vi "create event queue.vi"(8 "error in":errorcluster, 10 "size":i32, 11 "module in":refnum<class "TBM module execution interface.lvclass">) -> (0 "error out":errorcluster, 3 "module out":refnum<class "TBM module execution interface.lvclass">)   [LabVIEW 2013, in "TBM module execution interface.lvclass"]
uses:
  TBM module execution interface.lvclass
  TBM module execution interface.lvclass/TBM module execution interface.ctl
  <vilib>/NI/Tag Bus/events/data bus events.lvlib
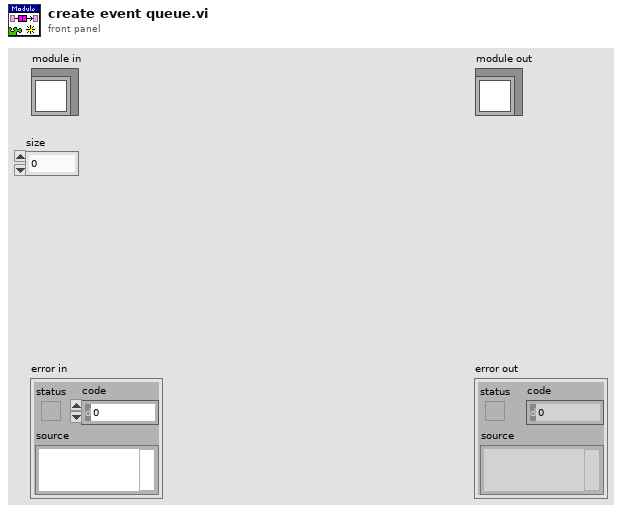
[diagram p1: front panel]
types:
  T1 = typedef "data bus events.lvlib/event queue.ctl" = cluster{"head":i32, "count":i32, "event array":T2[]}
  T2 = typedef "data bus events.lvlib/event.ctl" = cluster{"event group":i64, "event ID":i64, "int value":i64, "double value":dbl, "event time":timestamp}
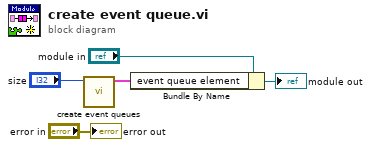
[diagram p0: block diagram]
diagram:
  n1 = call <vilib>:"create event queues.vi"("size"="size") -> ("event queue"=w2:T1)  [unwired: 10 in]
  n2 = Bundle By Name(cluster="module in", "event queue element"=w2) -> (→"module out":refnum<class "TBM module execution interface.lvclass">)
  "error out" <- "error in"
